vi "拉取依赖文件并更新.vi"(8 "error in (no error)":errorcluster, 11 "远端地址":string="/updatefiles/OneStation/V4/一体化微型水质监测站.zip") -> (0 "error out":errorcluster)   [LabVIEW 2016, in "update.lvlib" / "http client.lvclass"]
uses:
  http client.lvclass
  update.lvlib
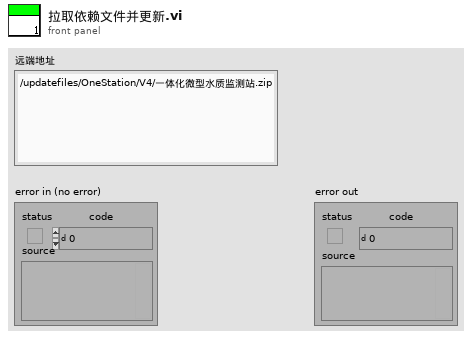
[diagram p1: front panel]
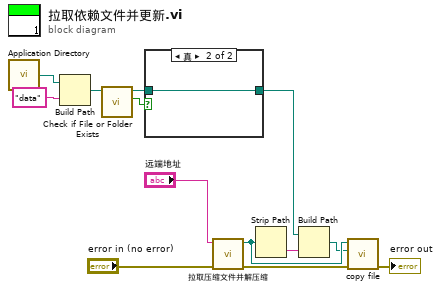
[diagram p0: block diagram]
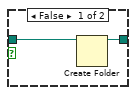
[diagram p2: hidden frame]
diagram:
  n1 = call <vilib>:"Application Directory.vi"() -> ("Application Directory"=w11:path)
  n2 = Build Path(base path=w11, name or relative path="data" ("名称或相对路径")) -> (appended path=w3:path)
  n3 = call <vilib>:"Check if File or Folder Exists.vi"("path"=w3) -> ("file or folder exists?"=w1:bool, "dup path"=w2:path)  [unwired: 8 in, 1 out]
  n4 = case shown="真" w1 {
    tunnel: w2 -> [w15 w16]
    tunnel: [w14 w16] -> w4
    frame False {
      n5 = Create Folder(path (use dialog)=w15) -> (created path=w14:path)  [unwired: 2 in, 2 out]
    }
    frame True {
    }
  }
  n6 = call "拉取压缩文件并解压缩.vi"("error in (no error)"="error in (no error)", "远端地址"="远端地址") -> ("error out"=w13:errorcluster, "文件路径"=w9:path)  [unwired: 8 in]
  n7 = Strip Path(path=w9) -> (name=w8:string)  [unwired: 1 out]
  n8 = Build Path(base path=w4, name or relative path=w8) -> (appended path=w7:path)
  n9 = call "copy file.vi"("error in (no error)"=w13, "目标路径（使用对话框）"=w7, "源路径"=w9) -> ("error out"=→"error out":errorcluster)  [unwired: 8 in]
